vi "ConnSNK3 (SubVI).vi"(8 "error in (no error)":errorcluster, 11 "String in":refnum<vi>) -> (0 "error out":errorcluster, 3 "conParam.TCP_conn":bool)   [LabVIEW 2017]
uses:
  Global_SNK3_HF.vi
  LV_Unicorn/LV_Unicorn.lvlib
panel:
  out "String":string
  # "Подключение к устройству"
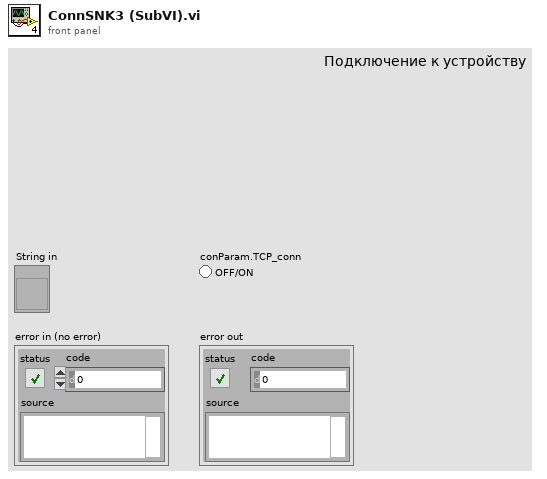
[diagram p1: front panel]
types:
  T1 = typedef "LV_Unicorn.lvlib/unicorn_Param.ctl" = cluster{"conParam":T2, "Param":T3}
  T2 = typedef "LV_Unicorn.lvlib/unicorn_conn.ctl" = cluster{"ReadIntParam":bool, "ReadDescrParam":bool, "ReadFloatParam":bool, "debug":bool, "ReadJSON":bool, "IP_address":string, "N_attempts":i32, "type_con":enum16{"Serial", "TCP"}, "MB_address":i32, "VISA":refnum<visa-resource-name>, "connection ID":refnum<k5>, "nameDevices":string, "timeout":i32, "port":u16, "type_version":string, "baud_rate":u32, "VersionControl":bool, "TCP_conn":bool, "WindowSize":i32}
  T3 = typedef "LV_Unicorn.lvlib/unicorn_JSON.ctl" = cluster{"NumParam":cluster{"NTelem":i32, "NInt":i32, "NFloat":i32, "NTable":i32}, "ParamInt":T4, "Telemetry":T5, "Table":T6, "ParamFloat":T7}
  T4 = typedef "LV_Unicorn.lvlib/unicorn_ParamInt.ctl" = cluster{"ID":string, "Num":i32, "Name":string, "Type":string, "Enum":string, "Desc":string, "Unit":string, "Access":string, "FormatStr":string, "Min":i32, "Max":i32}[]
  T5 = typedef "LV_Unicorn.lvlib/unicorn_Telemetry.ctl" = cluster{"ID":string, "Num":i32, "Name":string, "Desc":string, "Unit":string, "FormatStr":string, "Min":i32, "Max":i32}[]
  T6 = typedef "LV_Unicorn.lvlib/unicorn_Table.ctl" = cluster{"Num":i32, "Access":string, "ColumnCount":i32, "NeedParamPrepare":bool, "Columns":cluster{"Column":i32, "Desc":string, "Name":string}[], "DataType":string, "FormatStr":string, "ID":string, "Name":string, "RowCount":i32, "Rows":cluster{"Desc":string, "ID":string, "Max":i32, "Min":i32, "Name":string, "Row":i32, "Unit":string}[], "Type":string}[]
  T7 = typedef "LV_Unicorn.lvlib/unicorn_ParamFloat.ctl" = cluster{"ID":string, "Num":i32, "Name":string, "Type":string, "Enum":string, "Desc":string, "Unit":string, "Access":string, "FormatStr":string, "Min":sgl, "Max":sgl}[]
  T8 = typedef "LV_Unicorn.lvlib/unicorn_array.ctl" = cluster{"ArrayInt":i32[], "ArrayFloat":sgl[], "Telemetry":sgl[], "ArrayIntStr":string[][], "ArrayFloatStr":string[][], "ArrayTelemetryStr":string[][]}
  T9 = typedef "OptionPACK5.ctl" = cluster{"MagicWordStr":string, "Header size":u32, "Проверка CRC8":bool, "Проверка конца пакета":bool, "GainCompens":bool, "Неотбрасывать BadEnd пакеты":bool, "Неотбрасывать BadCRC пакеты":bool, "Привести к 1":bool, "GainCoef":bool, "K_scale":dbl, "ScaleOrdinate":enum16{"Отсчеты АЦП (±32767)", "Проценты", "Вольты", "дБмкВ (отн. 1 мкВ)", "Отсчеты АЦП (±1)"}}
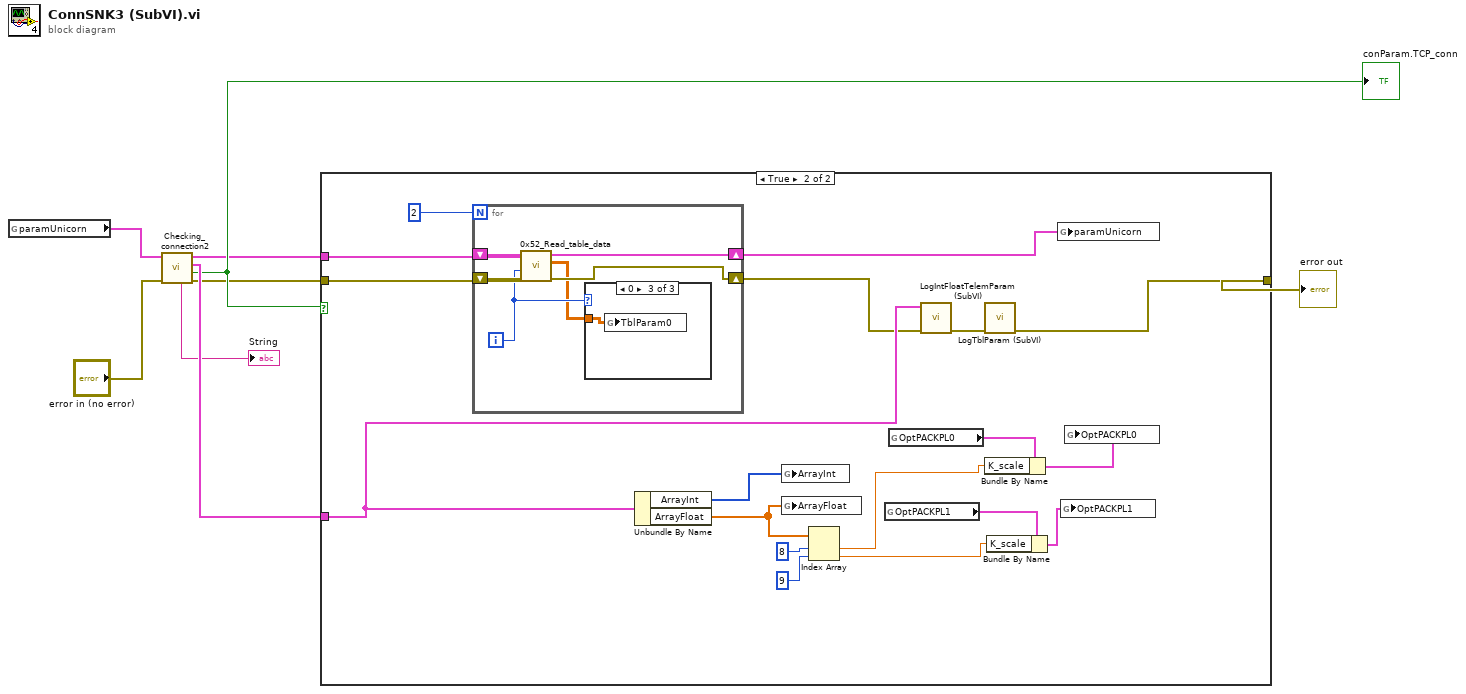
[diagram p0: block diagram]
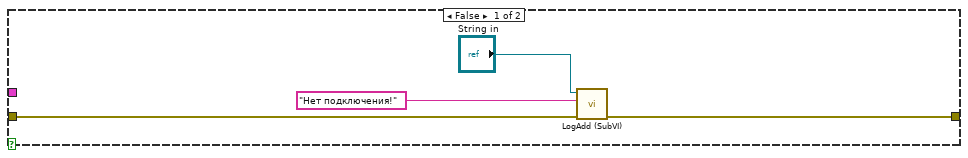
[diagram p2: hidden frame]
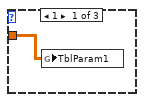
[diagram p3: hidden frame]
diagram:
  n1 = global read "Global_SNK3_HF.vi" "paramUnicorn"() -> (w3:T1)
  n2 = call "Checking_connection2.vi"("error in"="error in (no error)", "paramUnicornIn"=w3) -> ("error out"=w2:errorcluster, "conParam.TCP_conn"=w5:bool, "ArrayData"=w6:T8, "paramUnicorn"=w4:T1, "Описание устройства"=→"String":string)  [unwired: 4 in, 1 out]
  "conParam.TCP_conn" <- w5
  n3 = case shown="True" w5 {
    tunnel: w2 -> [w10 w17]
    tunnel: w4 -> [_ w18]
    tunnel: w6 -> [_ w15]
    tunnel: [w9 w16] -> w7
    frame False {
      n4 = call "LogAdd (SubVI).vi"("error in"=w10, "string"="Нет подключения!", "Log"="String in") -> ("error out"=w9:errorcluster)  [unwired: 8 in]
    }
    frame True {
      n5 = for {
        N: 2 -> [_]
        shift-right: [w33] -> w29
        shift-left: w18 -> [w36]
        shift-right: [w32] -> w14
        shift-left: w17 -> [w34]
        i -> [w35]
        n6 = call "0x52_Read_table_data.vi"("error in"=w34, "NTable"=w35, "paramUnicornIn"=w36) -> ("error out"=w32:errorcluster, "Array"=w31:sgl[][], "paramUnicornOut"=w33:T1)  [unwired: 6 in]
        n7 = case shown="0" w35 {
          tunnel: w31 -> [w37 _ w38]
          frame 1 {
            n8 = global write "Global_SNK3_HF.vi" "TblParam1"(w37) -> ()
          }
          frame 2, Default {
          }
          frame 0 {
            n9 = global write "Global_SNK3_HF.vi" "TblParam0"(w38) -> ()
          }
        }
      }
      n10 = Unbundle By Name(w15) -> ("ArrayInt"=w20:i32[], "ArrayFloat"=w19:sgl[])
      n11 = global write "Global_SNK3_HF.vi" "ArrayInt"(w20) -> ()
      n12 = global write "Global_SNK3_HF.vi" "ArrayFloat"(w19) -> ()
      n13 = Index Array(array=w19, index #1=8 ("index"), index #2=9 ("index")) -> (element #1=w22:sgl, element #2=w21:sgl)
      n14 = global read "Global_SNK3_HF.vi" "OptPACKPL1"() -> (w26:T9)
      n15 = global read "Global_SNK3_HF.vi" "OptPACKPL0"() -> (w28:T9)
      n16 = call "LogIntFloatTelemParam (SubVI).vi"("error in"=w14, "ArrayData"=w15) -> ("error out"=w13:errorcluster)  [unwired: 9 in]
      n17 = call "LogTblParam (SubVI).vi"("error in"=w13) -> ("error out"=w16:errorcluster)  [unwired: 10 in]
      n18 = Bundle By Name(cluster=w28, "K_scale"=w22) -> (w27:T9)
      n19 = Bundle By Name(cluster=w26, "K_scale"=w21) -> (w25:T9)
      n20 = global write "Global_SNK3_HF.vi" "paramUnicorn"(w29) -> ()
      n21 = global write "Global_SNK3_HF.vi" "OptPACKPL1"(w25) -> ()
      n22 = global write "Global_SNK3_HF.vi" "OptPACKPL0"(w27) -> ()
    }
  }
  "error out" <- w7
